vi "ENPH 354 Assignment 2 - Q1 .vi"() -> ()   [LabVIEW 2021]
panel:
  in  "stop":bool
  out "Waveform Chart":cluster{dbl, "number: 0 to 1":dbl}(graph)
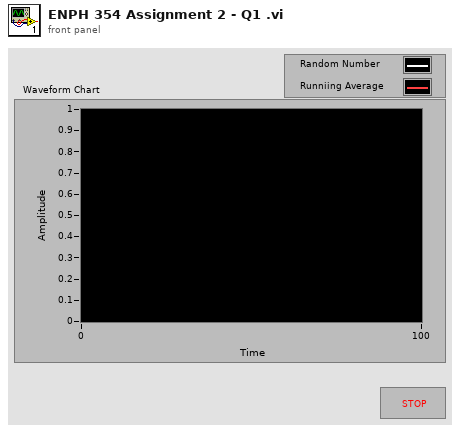
[diagram p1: front panel]
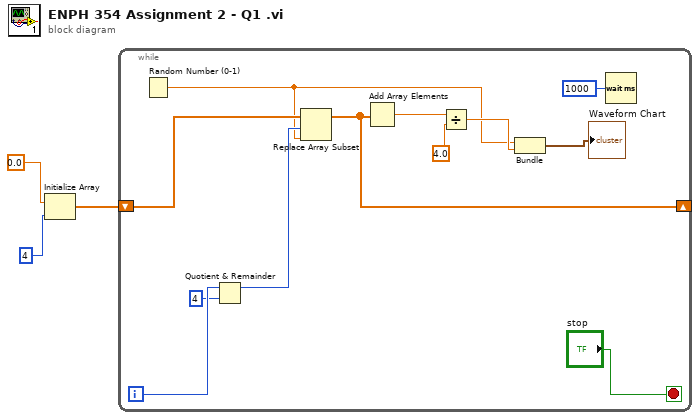
[diagram p0: block diagram]
diagram:
  n1 = Initialize Array(0.0 ("element"), 4 ("dimension size")) -> (w1:dbl[])
  n2 = while {
    shift-right: [w8] -> _
    shift-left: w1 -> [w14]
    i -> [w13]
    stop <- "stop" stop-if-true
    n3 = Random Number (0-1)() -> (number: 0 to 1=w4:dbl)
    n4 = Quotient & Remainder(x=w13, y=4) -> (x-y*floor(x/y)=w11:i32)  [unwired: 1 out]
    n5 = Replace Array Subset(array=w14, new element=w4, index=w11) -> (w8:dbl[])
    n6 = Add Array Elements(numeric array=w8) -> (sum=w10:dbl)
    n7 = Divide(x=w10, y=4.0) -> (x/y=w5:dbl)
    n8 = Bundle("number: 0 to 1"=w4, w5) -> (→"Waveform Chart":cluster{"number: 0 to 1":dbl, dbl})  [unwired: 1 in]
    n9 = Wait (ms)(milliseconds to wait=u32 1000) -> ()  [unwired: 1 out]
  }
